vi "TemperatureTest.vi"() -> ()   [LabVIEW 2017]
uses:
  <instrlib>/Mercury iXX/Public/Controls/Comms Transport Layer.ctl
  <instrlib>/Mercury iXX/Public/Controls/Unit String.ctl
  <instrlib>/Mercury iXX/Public/Libraries/System/Open/Open System.vi
  <instrlib>/Mercury iXX/Public/Libraries/System/Read/Catalogue (Read).vi
  <instrlib>/Mercury iXX/Public/Libraries/Temperature/Open/Open Temperature Device.vi
  <instrlib>/Mercury iXX/Public/Libraries/Temperature/Signals/Read/Temperature (Read).vi
  <instrlib>/Mercury iXX/Mercury iXX.lvlib
  <instrlib>/Mercury iXX/Public/Libraries/Temperature.lvlib
  <instrlib>/Mercury iXX/Public/Libraries/System.lvlib
panel:
  out "Array":string[](array[string])
  out "Array 2":string[](array[string])
  out "Temperature":dbl
  out "Unit":T1
  in  "Stop":bool
  in  "Read Interval (s)":sgl=1.0 min=0.25 max=1000 step=0.25 format="%.2f"
  out "error out":errorcluster
  in  "Device Identifier":string="MB1.T1:TEMP"
  in  "Comms Layer":T2
  in  "VISA resource name":refnum<visa-resource-name>
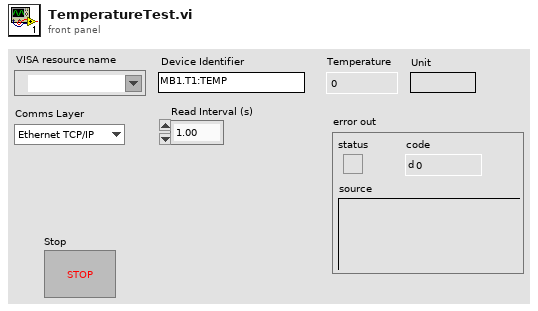
[diagram p1: front panel]
types:
  T1 = typedef "Mercury iXX.lvlib/Unit String.ctl" = string
  T2 = typedef "Mercury iXX.lvlib/Comms Transport Layer.ctl" = enum16{"Ethernet TCP/IP", "USB", "ISOBus - RS-232", "GPIB"}
  T3 = typedef "Mercury iXX.lvlib/Mercury Reference.ctl" = cluster{"Comms":refnum<visa-resource-name>, "Device ID":string[], "Comms Layer":T2, "Command":string, "Query reference":T4}
  T4 = typedef "Mercury iXX.lvlib/Query Dynamic Reference.ctl" = refnum<vi>
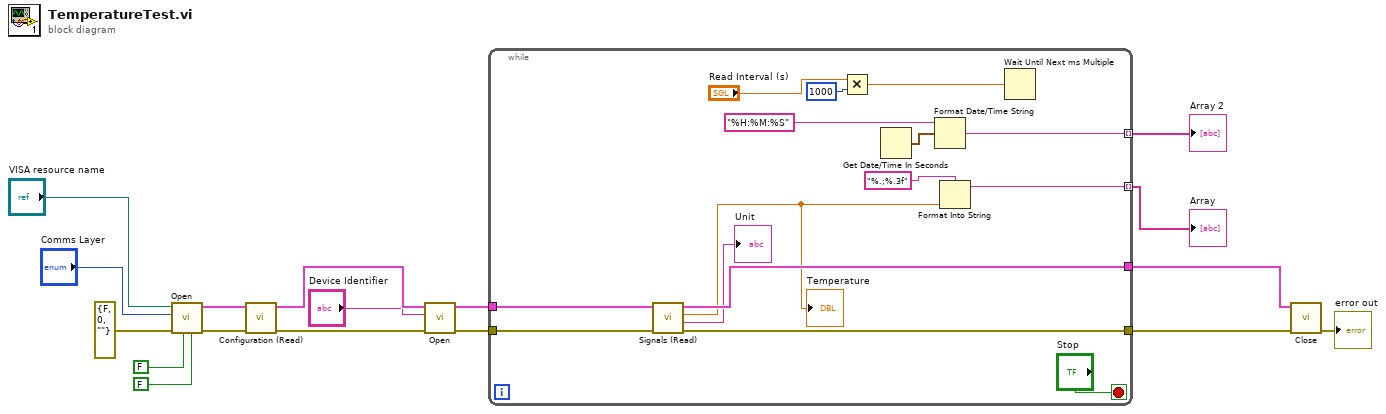
[diagram p0: block diagram]
diagram:
  n1 = call-poly <instrlib>:"Open.vi"("Clear Previous Connections (False)"=FALSE, "ID Query (True)"=FALSE, "error in (no error)"=errorcluster {"status"=FALSE, "code"=0, "source"=""}, "Comms Layer"="Comms Layer", "VISA resource name"="VISA resource name") -> ("error out"=w14:errorcluster, "Mercury Reference Out"=w15:T3)  [unwired: 2 in, 3 out]
  n2 = call-poly <instrlib>:"Configuration (Read).vi"("error in"=w14, "Mercury Reference In"=w15) -> ("error out"=w12:errorcluster, "Mercury Reference Out"=w13:T3)  [unwired: 6 in, 2 out]
  n3 = call-poly <instrlib>:"Open.vi"("error in (no error)"=w12, "Device Identifier"="Device Identifier", "Mercury Reference In"=w13) -> ("error out"=w9:errorcluster, "Mercury Reference Out"=w10:T3)  [unwired: 7 in]
  n4 = while {
    tunnel: w10 -> [w32]
    tunnel: w9 -> [w31]
    tunnel: [w30] -> w8
    tunnel: [w29] -> w7
    tunnel: [w18] -> w1 mode=indexing
    tunnel: [w21] -> w2 mode=indexing
    stop <- "Stop" stop-if-true
    n5 = call-poly <instrlib>:"Signals (Read).vi"("error in"=w31, "Mercury Reference In"=w32) -> ("error out"=w30:errorcluster, "Unit"=→"Unit":T1, "Temperature"=w19:dbl, "Mercury Reference Out"=w29:T3)  [unwired: 5 in, 1 out]
    "Temperature" <- w19
    n6 = Multiply(x="Read Interval (s)", y=u32 1000 ("millisecond multiple")) -> (x*y=w24:sgl)
    n7 = Get Date/Time In Seconds() -> (seconds since 1Jan1904=w22:timestamp)
    n8 = Format Date/Time String(time format string (%c)="%H:%M:%S", seconds (now)=w22) -> (date/time string=w21:string)  [unwired: 1 in]
    n9 = Format Into String(format string="%.;%.3f", w19) -> (resulting string=w18:string)  [unwired: 2 in, 1 out]
    n10 = Wait Until Next ms Multiple(millisecond multiple=w24) -> ()  [unwired: 1 out]
  }
  "Array 2" <- w2
  "Array" <- w1
  n11 = call <instrlib>:"Close.vi"("error in (no error)"=w8, "Mercury Reference"=w7) -> ("error out"=→"error out":errorcluster)  [unwired: 9 in]
